vi "Kinematic_Globals.vi"() -> ()   [LabVIEW 2018]
panel:
  in  "Max_Rotational_Speed":dbl
  in  "Max_Linear_Speed":dbl
  in  "Wheel_Circumference":dbl
  in  "Wheel_Diameter":dbl
  in  "Max_Wheel_Speed":dbl
  in  "Y_Offset":dbl
  in  "X_Offset":dbl
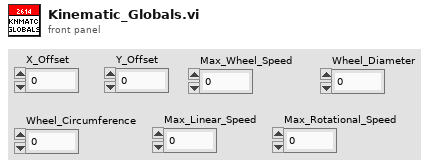
[diagram p1: front panel]
diagram:
